vi "pwm_interface_test.vi"() -> ()   [LabVIEW 2013]
panel:
  out "Numeric":i32
  out "status":string
  in  "low times":dbl format="%#_13g"
  in  "pulse number":i32
  in  "high times":dbl format="%#_13g"
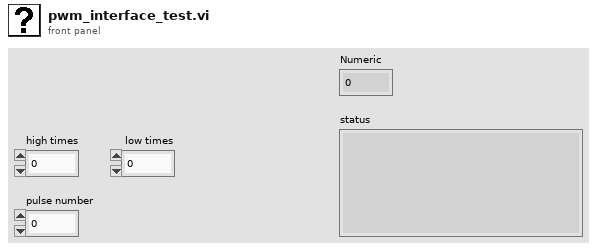
[diagram p1: front panel]
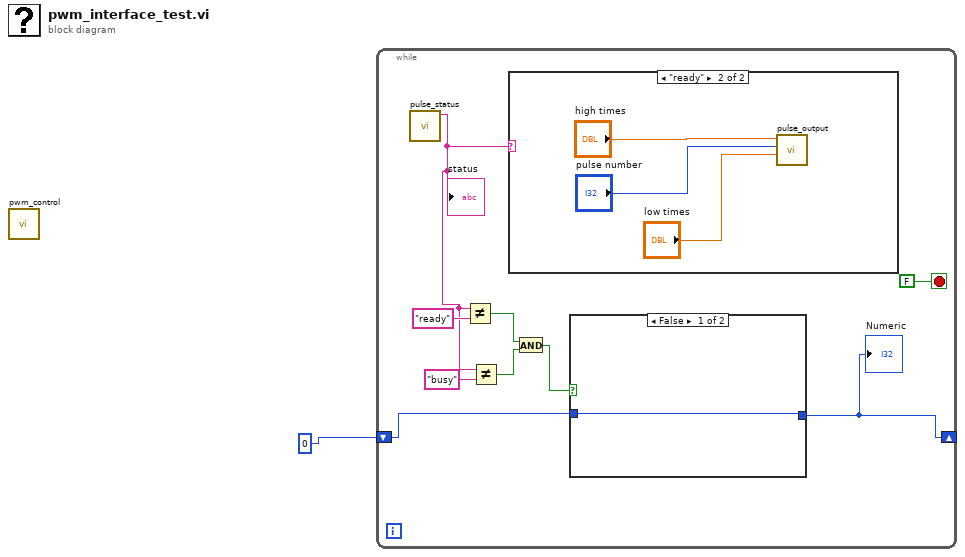
[diagram p0: block diagram]
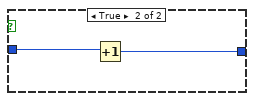
[diagram p2: hidden frame]
diagram:
  n1 = call "pwm_control.vi"() -> ()  [unwired: 11 in, 1 out]
  n2 = while {
    shift-right: [w2] -> _
    shift-left: 0 -> [w3]
    stop <- FALSE stop-if-true
    n3 = call "pulse_status.vi"() -> ("status"=w8:string)  [unwired: 10 in, 1 out]
    "status" <- w8
    n4 = Not Equal?(x=w8, y="ready") -> (x != y?=w6:bool)
    n5 = Not Equal?(x=w8, y="busy") -> (x != y?=w5:bool)
    n6 = case shown="\"ready\"" w8 {
      frame "False", Default {
      }
      frame "ready" {
        n7 = call "pulse_output.vi"("low times"="low times", "pulse number"="pulse number", "high times"="high times") -> ()  [unwired: 8 in, 1 out]
      }
    }
    n8 = And(x=w6, y=w5) -> (x .and. y?=w4:bool)
    n9 = case shown="False" w4 {
      tunnel: w3 -> [w11 w13]
      tunnel: [w11 w12] -> w2
      frame False {
      }
      frame True {
        n10 = Increment(x=w13) -> (x+1=w12:i32)
      }
    }
    "Numeric" <- w2
  }
